vi "HitrapGUI.HTLE_TR5.vi"() -> ()   [LabVIEW 2014, in "HitrapGUI.lvlib"]
uses:
  HitrapGUI.lvlib
  CSlibraries/GUILib/GUILib.userEventsMainType.ctl
  CSlibraries-extern/DimLVEvent/DimIndicators/DimIndicators.anyType.ctl
  CSlibraries/GUILib/GUILib.simpleNumeric.ctl
  CSlibraries/GUILib/GUILib.basicNumeric.ctl
  CSlibraries-extern/DimLVEvent/DimIndicators/DimIndicators.numericType.ctl
  CSlibraries/UtilityLib/UtilityLib.valueStatus.ctl
  CS_Core/CSSystem/CoreDefs/CoreDefs.rawDataType.ctl
  CS_Core/CSSystem/CoreLib/CoreLib.double 2 byte array.vi
  CS_Core/CSSystem/CoreLib/CoreLib.int 2 byte array.vi
  CSlibraries/UtilityLib/UtilityLib.lvlib
  CS_Core/CSSystem/CSSystemLib/CSSystemLib.lvlib
  CSlibraries-extern/DimLVEvent/DimIndicators/DimIndicators.lvlib
  CS_Core/GUIs/GOGControllerGUI/GOGControllerGUI.lvlib
  CSlibraries/GUILib/GUILib.lvlib
  CS_Core/CSSystem/CoreLib/CoreLib.lvlib
  CSlibraries-extern/DimLVEvent/LVDimInterface/LVDimInterface.lvlib
panel:
  in  "MotorActivityLink-Act":T1
  in  "MotorLink-Act":T1
  in  "TR5DK1Link":T2
  in  "TR5DK2Link":T2
  in  "TR5DK1Ctl":T3 caption="TR5DK1" {"Progress Slide" scale=0.0..100.0; "Nom_Position" items=["Undefined", "Open", "Faraday Cup", "MCP"]}
  in  "TR5DK2Ctl":T3 caption="TR5DK2" {"Progress Slide" scale=0.0..100.0; "Nom_Position" items=["Undefined", "Open", "Faraday Cup", "MCP"]}
  in  "userEventsMain 2":T4
  in  "Next":bool
  in  "EnAn_TOF":bool=TRUE
  in  "EnAn_LEBT2":bool=TRUE
  in  "EnAn_LEBT1":bool=TRUE
  in  "EnAn_RFQ":bool=TRUE
  in  "EnAn_IH":bool=TRUE
  in  "EnAn_TOFCtl":T5 {"nom" step=1.0}
  in  "EnAn_LEBT2Ctl":T5 {"nom" step=1.0}
  in  "EnAn_LEBT1Ctl":T5 {"nom" step=1.0}
  in  "EnAn_RFQCtl":T5 {"nom" step=1.0}
  in  "EnAn_IHCtl":T5 {"nom" step=1.0}
  in  "TR3BB_2":bool=TRUE
  in  "TR3BB_1":bool=TRUE
  in  "TR3BB_2Ctl":T5 {"nom" step=1.0}
  in  "TR3BB_1Ctl":T5 {"nom" step=1.0}
  in  "TR5KY6Ctl":T5 {"nom" step=1.0}
  in  "TR5KX6Ctl":T5 {"nom" step=1.0}
  in  "TR5KY5Ctl":T5 {"nom" step=1.0}
  in  "TR5KX5Ctl":T5 {"nom" step=1.0}
  in  "TR5KY4Ctl":T5 {"nom" step=1.0}
  in  "TR5KX4Ctl":T5 {"nom" step=1.0}
  in  "TR5ME6Ctl":T5 {"nom" step=1.0}
  in  "TR5ME5Ctl":T5 {"nom" step=1.0}
  in  "TR5ME4Ctl":T5 {"nom" step=1.0}
  in  "TR5KY6":bool=TRUE
  in  "TR5KX6":bool=TRUE
  in  "TR5ME6":bool=TRUE
  in  "TR5ME5":bool=TRUE
  in  "TR5KY5":bool=TRUE
  in  "TR5KX5":bool=TRUE
  in  "TR5ME4":bool=TRUE
  in  "TR5KY4":bool=TRUE
  in  "TR5KX4":bool=TRUE
  in  "TR5ME3":bool=TRUE
  in  "TR5KY3":bool=TRUE
  in  "TR5KX3":bool=TRUE
  in  "TR5ME3Ctl":T5 {"nom" step=1.0}
  in  "TR5KY3Ctl":T5 {"nom" step=1.0}
  in  "TR5KX3Ctl":T5 {"nom" step=1.0}
  in  "TR5ME2Ctl":T5 {"nom" step=1.0}
  in  "TR5KY2Ctl":T5 {"nom" step=1.0}
  in  "TR5KX2Ctl":T5 {"nom" step=1.0}
  in  "TR5KY1Ctl":T5 {"nom" step=1.0}
  in  "TR5KX1Ctl":T5 {"nom" step=1.0}
  in  "TR5ME1Ctl":T5 {"nom" step=1.0}
  in  "TR5ME2":bool=TRUE
  in  "TR5KY2":bool=TRUE
  in  "TR5KX2":bool=TRUE
  in  "TR5KY1":bool=TRUE
  in  "TR5KX1":bool=TRUE
  in  "TR5ME1":bool=TRUE
  out "subSystem1State":string
  in  "subSystem1":bool
  out "subSystem1StateQuality":string
  in  "subControllersIgnoredDIM":T1
  in  "iniData":string
  in  "stop":bool
  in  "dummy":bool
  in  "parentSystem":bool
  in  "userEvent":refnum<user-event>
  # "TR5"
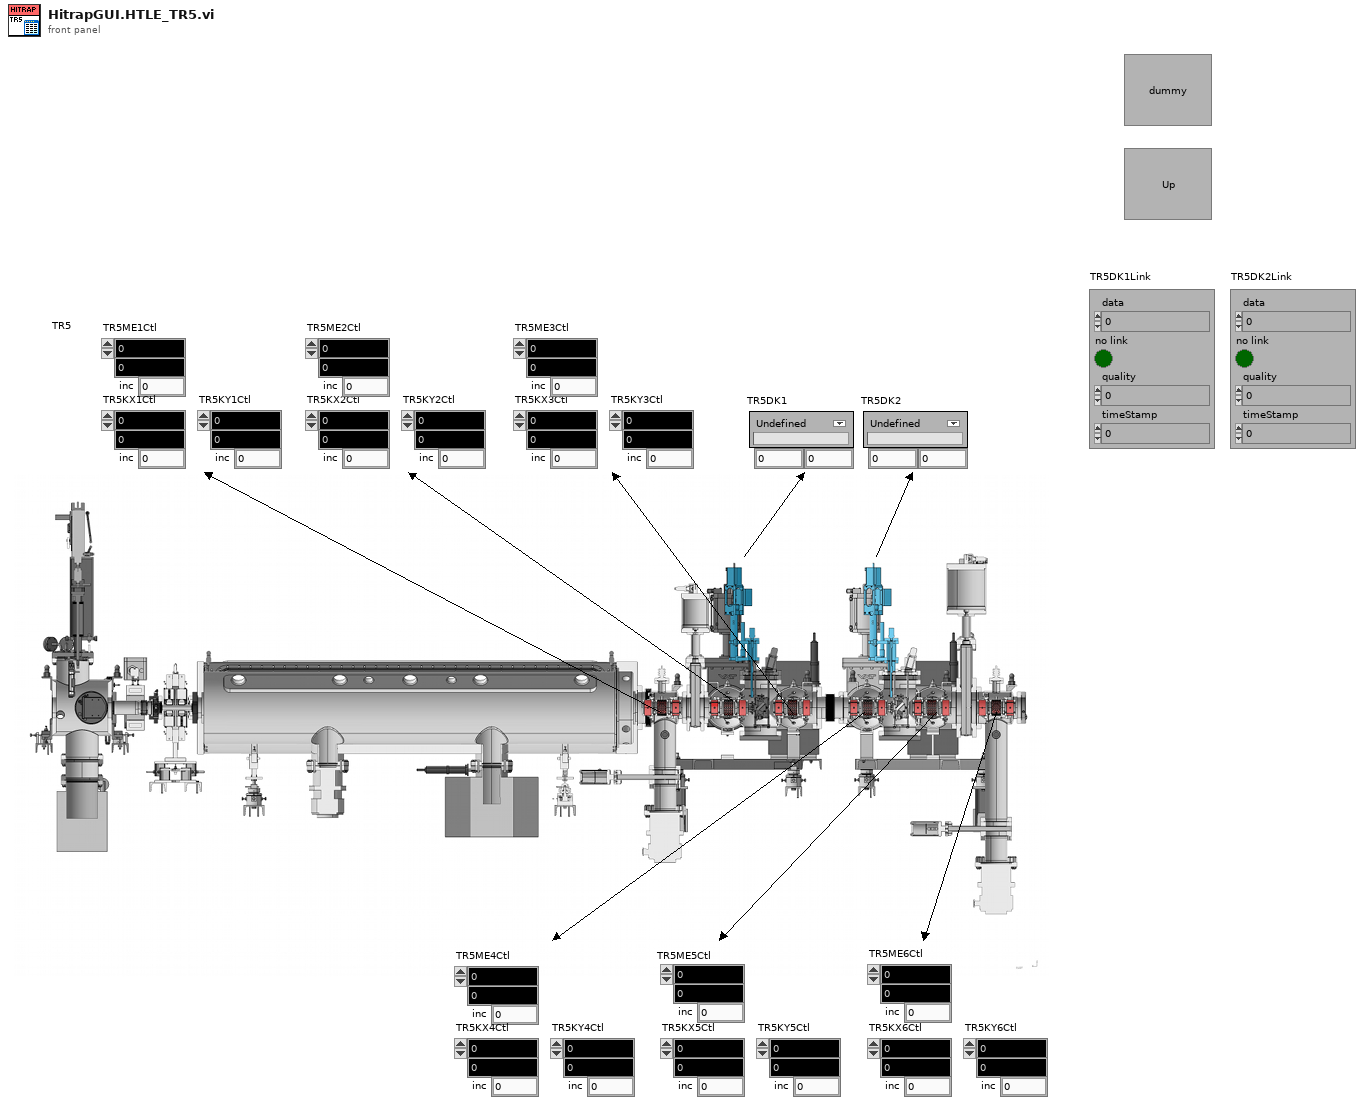
[diagram p1: front panel]
types:
  T1 = typedef "DimIndicators.lvlib/DimIndicators.anyType.ctl" = cluster{"data":string, "no link":bool, "quality":i32, "timeStamp":dbl}
  T2 = typedef "DimIndicators.lvlib/DimIndicators.numericType.ctl" = cluster{"data":dbl, "no link":bool, "quality":i32, "timeStamp":dbl}
  T3 = cluster{"Nom_Position":u8, "Progress Slide":u8, "TR6DK2Act":dbl, "TR6DK2Nom":dbl}
  T4 = typedef "GUILib.lvlib/GUILib.userEventsMainType.ctl" = cluster{"data":string, "dataType":i32}
  T5 = typedef "GUILib.lvlib/GUILib.simpleNumeric.ctl" = cluster{"nom":T6, "act":dbl, "inc":dbl}
  T6 = typedef "GUILib.lvlib/GUILib.basicNumeric.ctl" = dbl
  T7 = enum16{"Idle", "StartMotorActivity", "NewMotorDIM", "StopMotorActivity", "Stop"}
  T8 = typedef "UtilityLib.lvlib/UtilityLib.valueStatus.ctl" = enum16{"no info available", "stand by/off", "on", "warning", "alarm/malfunction", "not implemented", "user action required", "important information", "system default", "control default", "indicator default", "button default"}
  T9 = typedef "CoreDefs.rawDataType.ctl" = i8[]
  T10 = enum8{"Enabled", "Disabled", "Disabled and Grayed Out"}
  T11 = typedef "lveventtype.ctl" = enum32{"Null", "Timeout", "Annotation Menu Selection", "Annotation Menu Selection?", "App Instance Close", "App Instance Close?", "Autoscale Range Change", "Bookmark Info Change", "Cell Edit", "Cell Edit?", "Cursor Grab", "Cursor Grab?", "Cursor Menu Selection", "Cursor Menu Selection?", "Cursor Move", "Cursor Release", "Data Change", "Direction Change", "Display State Change", "Drag Ended", "Drag Enter", "Drag Leave", "Drag Over", "Drag Source Update", "Drag Starting", "Drag Starting?", "Drop", "Exec State Change", "Key Down", "Key Down?", "Key Repeat", "Key Repeat?", "Key Up", "Listbox Double Click", "Menu Activation?", "Menu Selection (App)", "Menu Selection? (App)", "Menu Selection (User)", "Mouse Down", "Mouse Down?", "Mouse Enter", "Mouse Leave", "Mouse Move", "Mouse Up", "Mouse Wheel", "NI Security User Change (App)", "Pane Size", "Panel Close", "Panel Close?", "Panel Resize", "Plot Attribute Change", "Scale Range Change", "Shortcut Menu Activation?", "Shortcut Menu Selection (App)", "Shortcut Menu Selection? (App)", "Shortcut Menu Selection (User)", "Tree Double Click", "Tree Drag", "Tree Drag?", "Tree Drop", "Tree Drop?", "Tree Item Close", "Tree Item Close?", "Tree Item Open", "Tree Item Open?", "User Event", "Value Change"}
  T12 = cluster{"TR5DK1Ctl":refnum<vi>, "byteArray out":T9}
  T13 = typedef "HitrapGUI.lvlib/HitrapGUI.i attribute.ctl" = cluster{"SVs":refnum<k21>[], "DSCIntProc":string, "MotorActivityID":i32}
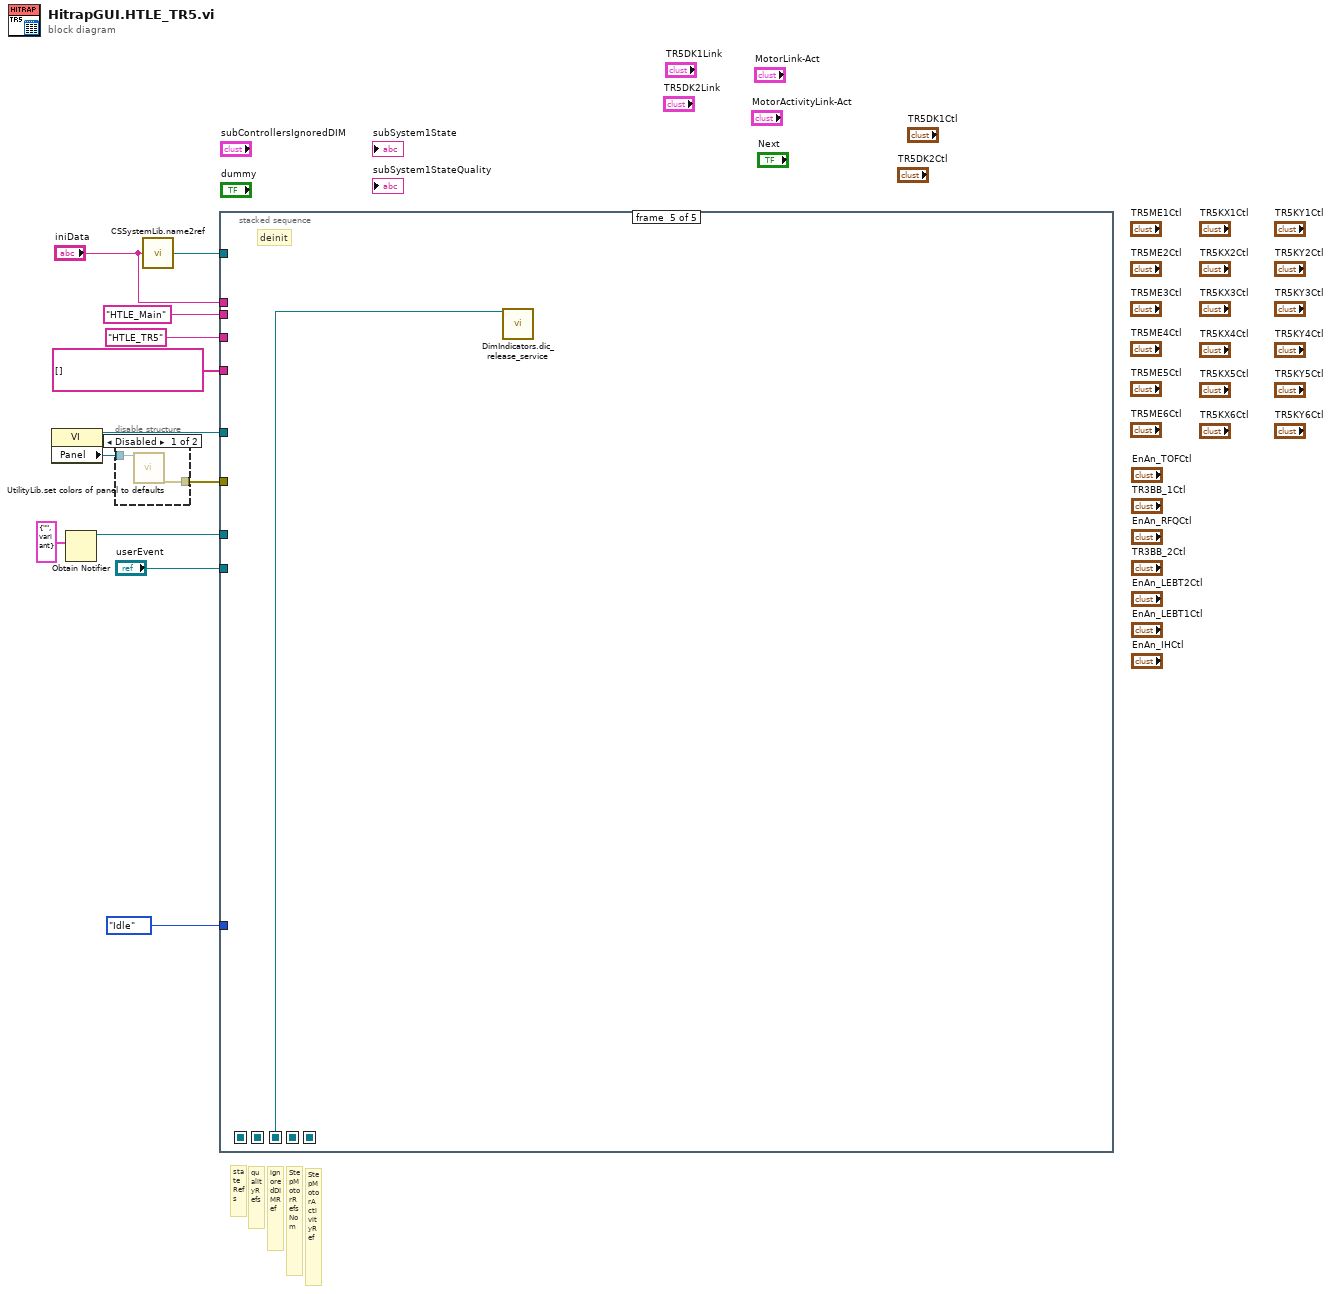
[diagram p0: block diagram]
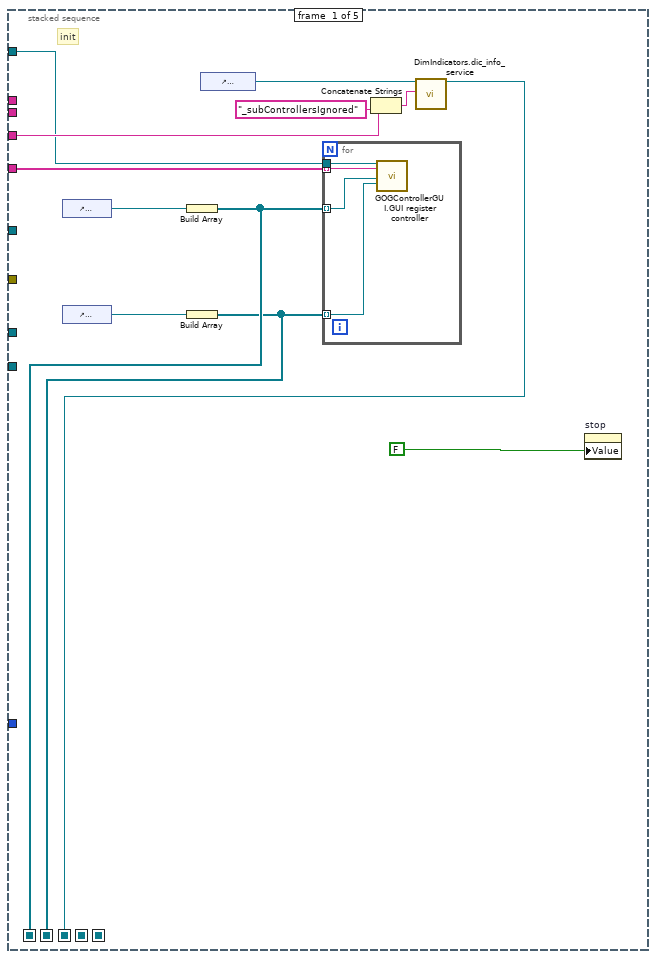
[diagram p3: hidden frame]
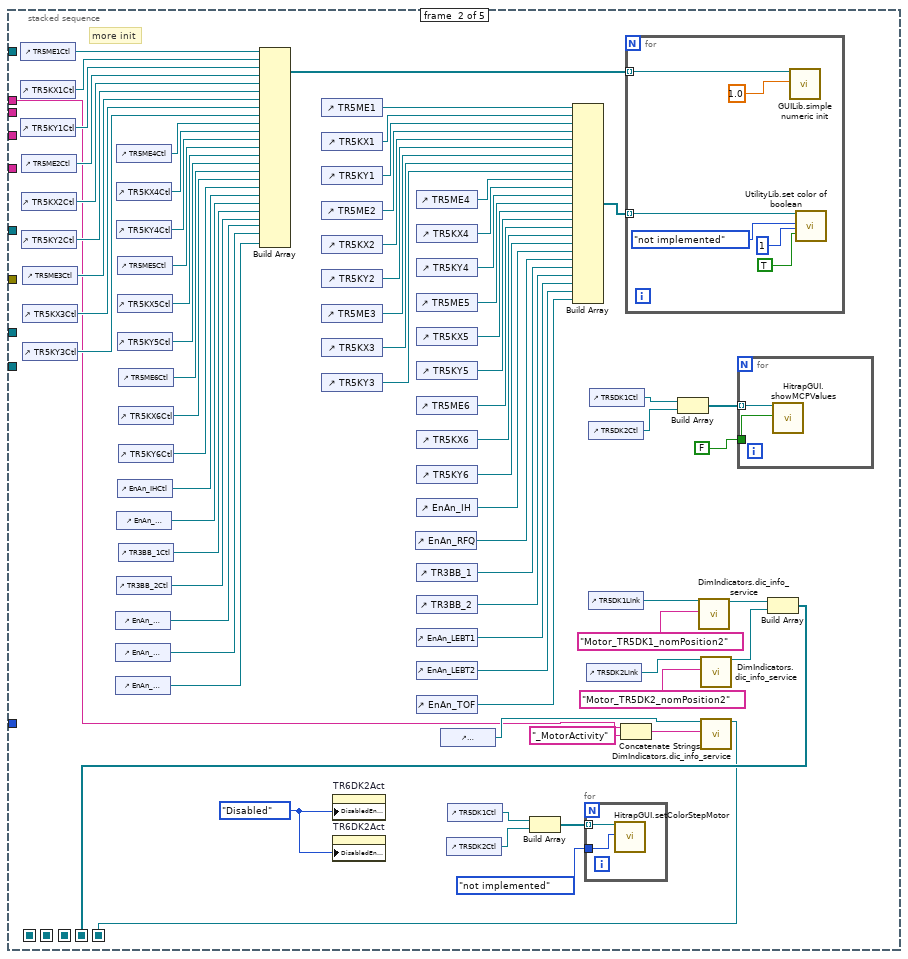
[diagram p4: hidden frame]
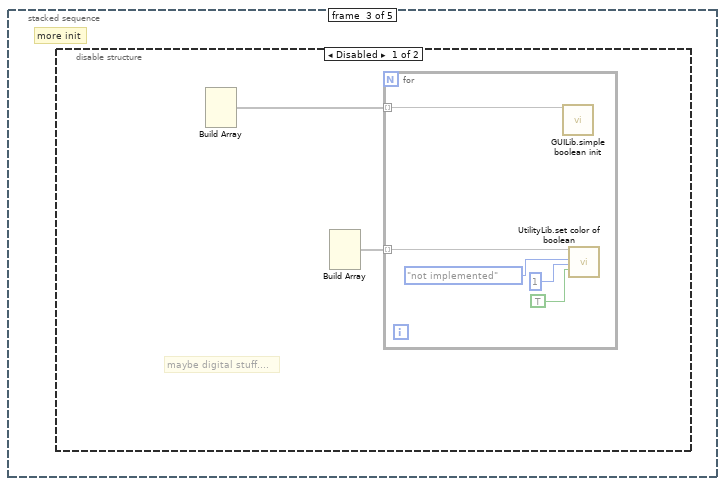
[diagram p5: hidden frame]
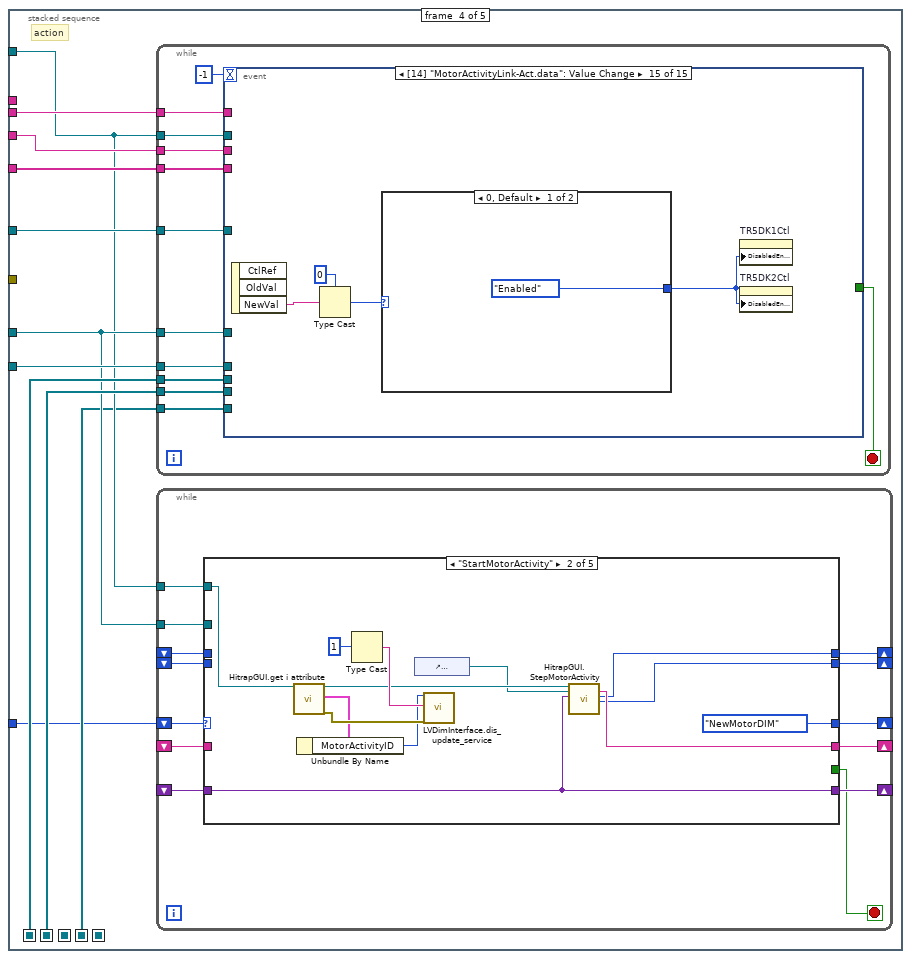
[diagram p7: hidden frame]
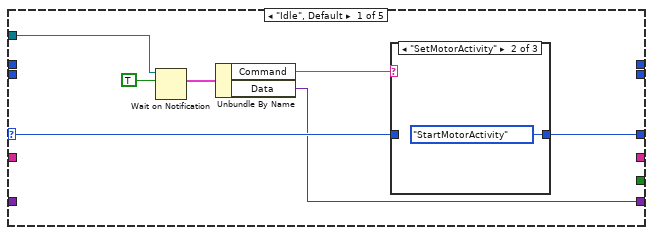
[diagram p8: hidden frame]
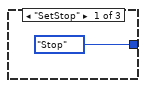
[diagram p9: hidden frame]
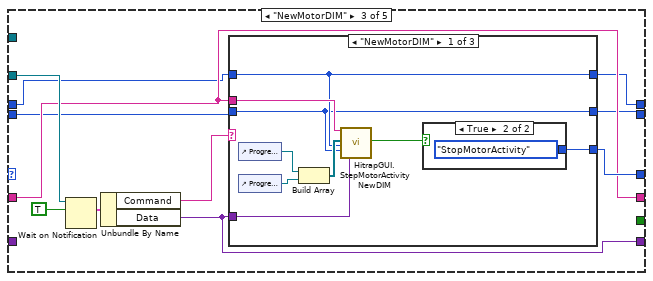
[diagram p11: hidden frame]
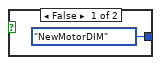
[diagram p12: hidden frame]
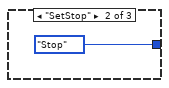
[diagram p13: hidden frame]
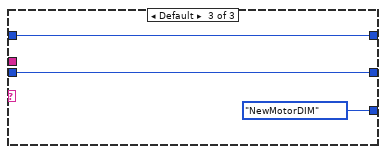
[diagram p14: hidden frame]
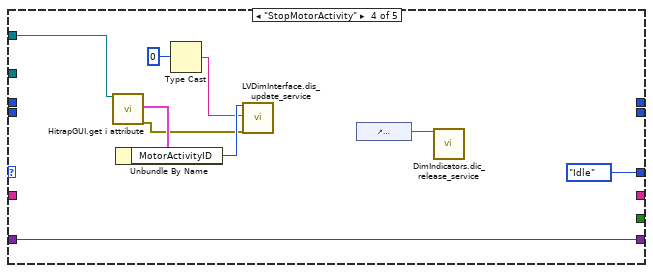
[diagram p15: hidden frame]
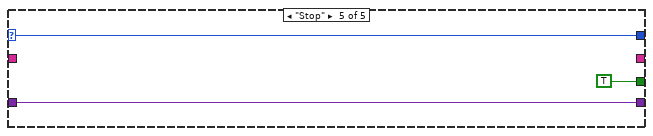
[diagram p16: hidden frame]
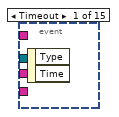
[diagram p17: hidden frame]
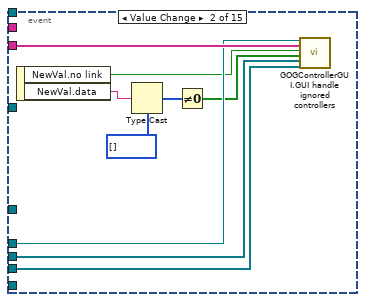
[diagram p18: hidden frame]
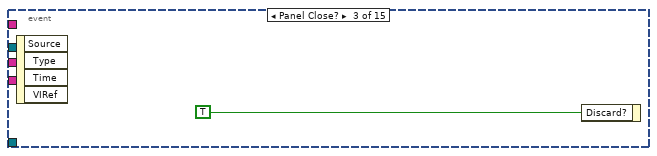
[diagram p19: hidden frame]
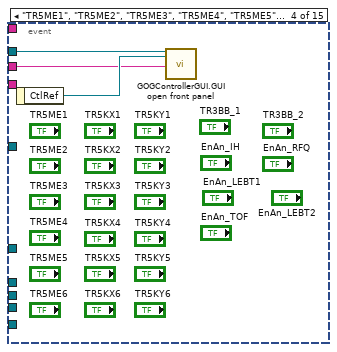
[diagram p20: hidden frame]
diagram:
  # "StepMotorActivityRef"
  # "StepMotorRefsNom"
  # "qualityRefs"
  # "ignoredDIMRef"
  # "stateRefs"
  n1 = property class="VI"() -> (reference out=w10:refnum<vi>, "Panel"=w11:refnum<vi>)  [unwired: 2 in, 1 out]
  n2 = Obtain Notifier(notification data type=cluster{"Command":string, "Data":variant} {"Command"="", "Data"=variant} ("EventData")) -> (notifier out=w2:refnum<notifier>)  [unwired: 3 in, 2 out]
  n3 = disable-structure shown="Disabled" {
    disable-tunnel: w11 -> [w14 _]
    disable-tunnel: [w13 _] -> w9
    frame Disabled {
      n4 = call "UtilityLib.set colors of panel to defaults.vi"("Front Panel"=w14) -> ("error out"=w13:errorcluster)  [unwired: 18 in]
    }
    frame Enabled {
    }
  }
  n5 = call "CSSystemLib.name2ref.vi"("name"="iniData") -> ("obj refnum"=w6:refnum<vi>)
  n6 = stacked-sequence {
    seq-local: [w16 _ _ _ _] -> [_ _ _ _ w346]
    seq-local: [w17 _ _ _ _] -> [_ _ _ w138 _]
    seq-local: [w15 _ _ _ _] -> [_ _ _ w137 _]
    seq-local: [_ w37 _ _ _] -> [_ _ _ w132 _]
    seq-local: [_ w36 _ _ _] -> [_ _ _ _ _]
    tunnel: "userEvent" -> [_ _ _ w141 _]
    tunnel: w10 -> [_ _ _ w140 _]
    tunnel: w9 -> [_ _ _ _ _]
    tunnel: "HTLE_TR5" -> [w22 _ _ w136 _]
    tunnel: string[] [] -> [w21 _ _ w139 _]
    tunnel: w6 -> [w20 _ _ w133 _]
    tunnel: "HTLE_Main" -> [_ _ _ w135 _]
    tunnel: "iniData" -> [_ w38 _ _ _]
    tunnel: w2 -> [_ _ _ w134 _]
    tunnel: T7."Idle" -> [_ _ _ w131 _]
    frame #0 {
      # "init"
      n7 = control-ref of="dummySubSystemState"() -> (w19:refnum<vi>)
      n8 = control-ref of="dummySubSystemStateQuality"() -> (w18:refnum<vi>)
      n9 = Build Array(w19) -> (w17:refnum<vi>[])
      n10 = Build Array(w18) -> (w15:refnum<vi>[])
      n11 = control-ref of="subControllersIgnoredDIM"() -> (w23:refnum<vi>)
      n12 = for {
        tunnel: w17 -> [w30] mode=indexing
        tunnel: w21 -> [w28] mode=indexing
        tunnel: w15 -> [w27] mode=indexing
        tunnel: w20 -> [w29]
        n13 = call "GOGControllerGUI.GUI register controller.vi"("i ref in"=w29, "controllerName"=w28, "subSystemState"=w30, "subSystemStateQuality"=w27) -> ()  [unwired: 14 in, 2 out]
      }
      n14 = Concatenate Strings(w22, "_subControllersIgnored" ("string")) -> (w25:string)
      n15 = call "DimIndicators.dic_info_service.vi"("controlRef"=w23, "serviceName"=w25) -> ("controlRef out"=w16:refnum<vi>)  [unwired: 16 in, 1 out]
      n16 = property on="stop" class="Bool (strict)"("Value"=FALSE ("stop")) -> ()  [unwired: 2 in, 2 out]
    }
    frame #1 {
      w31 = T10."Disabled" ("Disabled")
      # "more init"
      n17 = control-ref of="TR5ME1Ctl"() -> (w103:refnum<vi>)
      n18 = control-ref of="TR5KX1Ctl"() -> (w102:refnum<vi>)
      n19 = control-ref of="TR5KY1Ctl"() -> (w101:refnum<vi>)
      n20 = control-ref of="TR5ME2Ctl"() -> (w96:refnum<vi>)
      n21 = control-ref of="TR5KX2Ctl"() -> (w95:refnum<vi>)
      n22 = control-ref of="TR5KY2Ctl"() -> (w94:refnum<vi>)
      n23 = control-ref of="TR5ME3Ctl"() -> (w93:refnum<vi>)
      n24 = control-ref of="TR5KX3Ctl"() -> (w92:refnum<vi>)
      n25 = control-ref of="TR5KY3Ctl"() -> (w91:refnum<vi>)
      n26 = control-ref of="EnAn_LEBT1Ctl"() -> (w57:refnum<vi>)
      n27 = control-ref of="EnAn_LEBT2Ctl"() -> (w56:refnum<vi>)
      n28 = control-ref of="EnAn_TOFCtl"() -> (w55:refnum<vi>)
      n29 = control-ref of="TR5ME4Ctl"() -> (w90:refnum<vi>)
      n30 = control-ref of="TR5KX4Ctl"() -> (w89:refnum<vi>)
      n31 = control-ref of="TR5KY4Ctl"() -> (w88:refnum<vi>)
      n32 = control-ref of="EnAn_RFQCtl"() -> (w64:refnum<vi>)
      n33 = control-ref of="TR3BB_2Ctl"() -> (w60:refnum<vi>)
      n34 = control-ref of="TR5ME5Ctl"() -> (w87:refnum<vi>)
      n35 = control-ref of="TR5KX5Ctl"() -> (w86:refnum<vi>)
      n36 = control-ref of="TR5KY5Ctl"() -> (w85:refnum<vi>)
      n37 = control-ref of="EnAn_IHCtl"() -> (w65:refnum<vi>)
      n38 = control-ref of="TR5ME6Ctl"() -> (w84:refnum<vi>)
      n39 = control-ref of="TR5KX6Ctl"() -> (w83:refnum<vi>)
      n40 = control-ref of="TR5KY6Ctl"() -> (w82:refnum<vi>)
      n41 = control-ref of="TR3BB_1Ctl"() -> (w61:refnum<vi>)
      n42 = Build Array(w103, w102, w101, w96, w95, w94, w93, w92, w91, w90, w89, w88, w87, w86, w85, w84, w83, w82, w65, w64, w61, w60, w57, w56, w55) -> (w100:refnum<vi>[])
      n43 = control-ref of="TR5ME1"() -> (w99:refnum<vi>)
      n44 = control-ref of="TR5KX1"() -> (w98:refnum<vi>)
      n45 = control-ref of="TR5KY1"() -> (w81:refnum<vi>)
      n46 = control-ref of="TR5ME2"() -> (w80:refnum<vi>)
      n47 = control-ref of="TR5KX2"() -> (w79:refnum<vi>)
      n48 = control-ref of="TR5KY2"() -> (w78:refnum<vi>)
      n49 = control-ref of="TR5ME3"() -> (w77:refnum<vi>)
      n50 = control-ref of="TR5KX3"() -> (w76:refnum<vi>)
      n51 = control-ref of="TR5KY3"() -> (w75:refnum<vi>)
      n52 = property on="TR6DK2Act" class="DigNum (strict)"("DisabledEnum"=w31) -> ()  [unwired: 2 in, 2 out]
      n53 = property on="TR6DK2Act" class="DigNum (strict)"("DisabledEnum"=w31) -> ()  [unwired: 2 in, 2 out]
      n54 = control-ref of="EnAn_RFQ"() -> (w62:refnum<vi>)
      n55 = control-ref of="TR5ME4"() -> (w74:refnum<vi>)
      n56 = control-ref of="TR5KX4"() -> (w73:refnum<vi>)
      n57 = control-ref of="TR5KY4"() -> (w72:refnum<vi>)
      n58 = control-ref of="TR5ME5"() -> (w71:refnum<vi>)
      n59 = control-ref of="TR5KX5"() -> (w70:refnum<vi>)
      n60 = control-ref of="TR5KY5"() -> (w69:refnum<vi>)
      n61 = control-ref of="TR5ME6"() -> (w68:refnum<vi>)
      n62 = control-ref of="TR5KX6"() -> (w67:refnum<vi>)
      n63 = control-ref of="TR5KY6"() -> (w66:refnum<vi>)
      n64 = control-ref of="EnAn_IH"() -> (w63:refnum<vi>)
      n65 = control-ref of="TR3BB_1"() -> (w59:refnum<vi>)
      n66 = control-ref of="TR3BB_2"() -> (w58:refnum<vi>)
      n67 = control-ref of="EnAn_LEBT1"() -> (w54:refnum<vi>)
      n68 = control-ref of="EnAn_LEBT2"() -> (w53:refnum<vi>)
      n69 = control-ref of="EnAn_TOF"() -> (w52:refnum<vi>)
      n70 = control-ref of="MotorActivityLink-Act"() -> (w39:refnum<vi>)
      n71 = control-ref of="TR5DK2Ctl"() -> (w32:refnum<vi>)
      n72 = control-ref of="TR5DK1Ctl"() -> (w33:refnum<vi>)
      n73 = Build Array(w33, w32) -> (w34:refnum<vi>[])
      n74 = Build Array(w99, w98, w81, w80, w79, w78, w77, w76, w75, w74, w73, w72, w71, w70, w69, w68, w67, w66, w63, w62, w59, w58, w54, w53, w52) -> (w97:refnum<vi>[])
      n75 = for {
        tunnel: w34 -> [w105] mode=indexing
        tunnel: UtilityLib.valueStatus."not implemented" ("State") -> [w104]
        n76 = call "HitrapGUI.setColorStepMotor.vi"("Cluster Refnum"=w105, "State"=w104) -> ()  [unwired: 16 in, 2 out]
      }
      n77 = control-ref of="TR5DK2Link"() -> (w40:refnum<vi>)
      n78 = control-ref of="TR5DK2Ctl"() -> (w48:refnum<vi>)
      n79 = control-ref of="TR5DK1Link"() -> (w41:refnum<vi>)
      n80 = control-ref of="TR5DK1Ctl"() -> (w49:refnum<vi>)
      n81 = Concatenate Strings(w38, "_MotorActivity" ("string")) -> (w46:string)
      n82 = for {
        tunnel: w100 -> [w113] mode=indexing
        tunnel: w97 -> [w109] mode=indexing
        n83 = call "GUILib.simple numeric init.vi"("ctlRef"=w113, "increment"=1.0) -> ()  [unwired: 16 in, 2 out]
        n84 = call "UtilityLib.set color of boolean.vi"("button"=w109, "valueStatus"=UtilityLib.valueStatus."not implemented", "nOfPair (0)"=1, "setTRUEColor (FALSE)"=TRUE) -> ()  [unwired: 15 in, 1 out]
      }
      n85 = Build Array(w49, w48) -> (w50:refnum<vi>[])
      n86 = call "DimIndicators.dic_info_service.vi"("controlRef"=w41, "serviceName"="Motor_TR5DK1_nomPosition2") -> ("controlRef out"=w42:refnum<vi>)  [unwired: 16 in, 1 out]
      n87 = call "DimIndicators.dic_info_service.vi"("controlRef"=w40, "serviceName"="Motor_TR5DK2_nomPosition2") -> ("controlRef out"=w45:refnum<vi>)  [unwired: 16 in, 1 out]
      n88 = call "DimIndicators.dic_info_service.vi"("controlRef"=w39, "serviceName"=w46) -> ("controlRef out"=w36:refnum<vi>)  [unwired: 16 in, 1 out]
      n89 = for {
        tunnel: w50 -> [w107] mode=indexing
        tunnel: FALSE ("Visible") -> [w106]
        n90 = call "HitrapGUI.showMCPValues.vi"("Cluster Refnum"=w107, "show"=w106) -> ()  [unwired: 16 in, 2 out]
      }
      n91 = Build Array(w42, w45) -> (w37:refnum<vi>[])
    }
    frame #2 {
      # "more init"
      n92 = disable-structure shown="Disabled" {
        frame Disabled {
          # "maybe digital stuff...."
          n93 = Build Array() -> (w120:void[], w125:dbl, w124:dbl, w123:dbl, w122:dbl, w121:dbl)
          n94 = Build Array() -> (w114:void[], w119:dbl, w118:dbl, w117:dbl, w116:dbl, w115:dbl)
          n95 = for {
            tunnel: w120 -> [w130] mode=indexing
            tunnel: w114 -> [w126] mode=indexing
            n96 = call "GUILib.simple boolean init.vi"("ctlRef"=w130) -> ()  [unwired: 17 in, 2 out]
            n97 = call "UtilityLib.set color of boolean.vi"("button"=w126, "valueStatus"=UtilityLib.valueStatus."not implemented", "nOfPair (0)"=1, "setTRUEColor (FALSE)"=TRUE) -> ()  [unwired: 15 in, 1 out]
          }
        }
        frame Enabled {
        }
      }
    }
    frame #3 {
      # "action"
      n98 = while {
        tunnel: w141 -> [w227]
        tunnel: w140 -> [w225]
        tunnel: w139 -> [w223]
        tunnel: w138 -> [w222]
        tunnel: w137 -> [w221]
        tunnel: w133 -> [w220]
        tunnel: w136 -> [w219]
        tunnel: w135 -> [w218]
        tunnel: w134 -> [w217]
        tunnel: w132 -> [w216]
        stop <- w224 stop-if-true
        n99 = event shown="[14] \"MotorActivityLink-Act.data\": Value Change" {
          selector: _ -> [_ _ _ _ _ _ _ _ _ _ _ _ _ _ _]
          dyn-events: _ -> [_ _ _ _ _ _ _ _ _ _ _ _ _ _ _]
          timeout: -1 -> [_ _ _ _ _ _ _ _ _ _ _ _ _ _ _]
          tunnel: w227 -> [_ w232 _ _ w241 w252 _ w261 w265 _ _ _ _ _ _]
          tunnel: w225 -> [_ _ _ _ _ _ _ _ _ _ _ _ _ _ _]
          tunnel: [_ _ _ _ _ _ _ _ _ "stop" _ _ _ _ _] -> w224
          tunnel: w223 -> [_ w233 _ _ _ w248 _ _ _ _ _ _ _ _ _]
          tunnel: w222 -> [_ w229 _ _ _ _ _ _ _ _ _ _ _ _ _]
          tunnel: w221 -> [_ w228 _ _ _ _ _ _ _ _ _ _ _ _ _]
          tunnel: w220 -> [_ _ _ w240 _ _ _ _ w269 _ _ _ _ _ _]
          tunnel: w219 -> [_ _ _ w238 _ _ _ w259 w263 _ _ _ _ _ _]
          tunnel: w218 -> [_ _ _ _ _ w247 _ _ _ _ _ _ _ _ _]
          tunnel: w217 -> [_ _ _ _ _ _ _ _ _ w270 _ _ w312 w332 _]
          tunnel: w216 -> [_ _ _ _ _ _ _ _ _ _ w277 _ _ _ _]
          event Timeout {
            n100 = event-data() -> ()  [unwired: 1 in, 2 out]
          }
          event Value Change {
            n101 = event-data() -> ("NewVal.no link"=w231:bool, "NewVal.data"=w234:string)  [unwired: 1 in]
            n102 = Type Cast(type=T9 [] ("Array"), x=w234) -> (*(type *) &x=w236:T9)
            n103 = Not Equal To 0?(x=w236) -> (x != 0?=w230:bool[])
            n104 = call "GOGControllerGUI.GUI handle ignored controllers.vi"("userEvent"=w232, "controllerNames"=w233, "NOLINK"=w231, "controllersIgnored"=w230, "stateRefs"=w229, "qualityRefs"=w228) -> ()  [unwired: 14 in]
          }
          event Panel Close? {
            n105 = event-data() -> ()  [unwired: 1 in, 4 out]
            n106 = event-data("Discard?"=TRUE) -> ()  [unwired: 1 in, 1 out]
          }
          event "TR5ME1", "TR5ME2", "TR5ME3", "TR5ME4", "TR5ME5", "TR5ME6", "TR5KX1", "TR5KX2", "TR5KX3", "TR5KX4", "TR5KX5", "TR5KX6", "TR5KY1", "TR5KY2", "TR5KY3", "TR5KY4", "TR5KY5", "TR5KY6", "EnAn_IH", "EnAn_RFQ", "TR3BB_1", "TR3BB_2", "EnAn_LEBT1", "EnAn_LEBT2", "EnAn_TOF": Value Change {
            n107 = event-data() -> ("CtlRef"=w239:refnum<vi>)  [unwired: 1 in]
            n108 = call "GOGControllerGUI.GUI open front panel.vi"("i ref in"=w240, "elementRef"=w239, "controller"=w238) -> ()  [unwired: 15 in, 2 out]
          }
          event "Next": Value Change {
            n109 = event-data() -> ()  [unwired: 1 in, 3 out]
            n110 = Bundle By Name(cluster="userEventsMain 2", "data"="HTLE_TR6BT1", "dataType"=0) -> (w245:T4)
            n111 = Generate User Event(user event=w241, event data cluster=w245) -> ()  [unwired: 2 in, 2 out]
          }
          event "subSystem1", "parentSystem": Value Change {
            n112 = event-data() -> ("CtlRef"=w250:refnum<vi>)  [unwired: 1 in]
            n113 = control-ref of="parentSystem"() -> (w249:refnum<vi>)
            n114 = control-ref of="subSystem1"() -> (w253:refnum<vi>)
            n115 = Build Array (concatenate)(w247, w248) -> (w246:string[])
            n116 = Build Array(w249, w253) -> (w251:refnum<vi>[])
            n117 = call "GOGControllerGUI.GUI set selected subcontroller.vi"("userEvent"=w252, "controllerNames"=w246, "controllerRefs"=w251, "controllerRef"=w250) -> ()  [unwired: 16 in]
          }
          event Value Change {
            n118 = event-data() -> ("CtlRef"=w255:refnum<vi>, "NewVal"=w254:dbl)  [unwired: 1 in]
            n119 = call "GUILib.simple numeric change increment.vi"("ctlRef"=w255, "increment"=w254) -> ()  [unwired: 16 in, 2 out]
          }
          event Mouse Enter; Mouse Leave {
            n120 = event-data() -> ("CtlRef"=w258:refnum<vi>, "Type"=w257:T11)  [unwired: 1 in]
            n121 = case shown="\"Mouse Enter\"" w257 {
              tunnel: [TRUE _] -> w256
              frame "Mouse Enter" {
              }
              frame Default {
              }
            }
            n122 = call "GUILib.simple numeric show increment.vi"("ctlRef"=w258, "show"=w256) -> ("error out"=w260:errorcluster)  [unwired: 16 in, 1 out]
            n123 = call "GOGControllerGUI.GUI set error.vi"("userEvent"=w261, "controller"=w259, "GUIError"=w260) -> ()  [unwired: 16 in, 1 out]
          }
          event Value Change {
            n124 = event-data() -> ("CtlRef"=w268:refnum<vi>, "NewVal"=w267:T6)  [unwired: 1 in]
            n125 = call-poly "CoreLib.data 2 byte array.vi"("f64"=w267) -> ("byteArray out"=w266:T9)  [unwired: 18 in]
            n126 = call "GOGControllerGUI.GUI set nominal value.vi"("i ref in"=w269, "nominalRef"=w268, "nominalData"=w266, "controller"=w263) -> ("error out"=w264:errorcluster)  [unwired: 14 in, 1 out]
            n127 = call "GOGControllerGUI.GUI set error.vi"("userEvent"=w265, "controller"=w263, "GUIError"=w264) -> ()  [unwired: 16 in, 1 out]
          }
          event "stop": Value Change {
            n128 = event-data() -> ()  [unwired: 1 in, 6 out]
            n129 = Bundle("SetStop", "Data"=variant) -> (w273:cluster{string, "Data":variant})  [unwired: 1 in]
            n130 = Send Notification(notification=w273, notifier=w270) -> ()  [unwired: 1 in, 2 out]
          }
          event Value Change {
            n131 = event-data() -> ("CtlRef"=w276:refnum<vi>, "NewVal.data"=w278:dbl, "NewVal.no link"=w275:bool)  [unwired: 1 in]
            n132 = case shown="-2" w278 {
              tunnel: [w306 -1.0] -> w280
              tunnel: w278 -> [w306 _]
              frame 0, Default {
              }
              frame -2 {
              }
            }
            n133 = Increment(x=w280) -> (x+1=w281:dbl)
            n134 = To Unsigned Byte Integer(number=w281) -> (unsigned 8bit integer=w279:u8)
            n135 = for {
              tunnel: w275 -> [w288]
              tunnel: w276 -> [w284]
              tunnel: w279 -> [w287]
              tunnel: w277 -> [w286] mode=indexing
              i -> [w289]
              w282 = 0
              n136 = Type Cast(type=w282, x=w286) -> (*(type *) &x=w285:i32)
              n137 = Type Cast(type=w282, x=w284) -> (*(type *) &x=w283:i32)
              n138 = Equal?(x=w283, y=w285) -> (x = y?=w290:bool)
              n139 = case shown="True" w290 {
                tunnel: w289 -> [_ w296]
                tunnel: w288 -> [_ w295]
                tunnel: w287 -> [_ w294]
                frame False {
                }
                frame True {
                  n140 = case shown="0" w296 {
                    tunnel: w294 -> [_ w303 w304]
                    tunnel: [_ w302 w305] -> w293
                    frame Default {
                    }
                    frame 0 {
                      n141 = property on="Nom_Position" class="Ring (strict)"("Value"=w303) -> ()  [unwired: 2 in, 2 out]
                      n142 = control-ref of="TR5DK1Ctl"() -> (w302:refnum<vi>)
                    }
                    frame 1 {
                      n143 = property on="Nom_Position" class="Ring (strict)"("Value"=w304) -> ()  [unwired: 2 in, 2 out]
                      n144 = control-ref of="TR5DK2Ctl"() -> (w305:refnum<vi>)
                    }
                  }
                  n145 = case shown="False" w295 {
                    tunnel: [w298 UtilityLib.valueStatus."not implemented" ("State")] -> w292
                    tunnel: TRUE -> [w297 _]
                    frame False {
                      n146 = case shown="False" w297 {
                        tunnel: [UtilityLib.valueStatus."warning" ("State") UtilityLib.valueStatus."on" ("State")] -> w298
                        frame False {
                        }
                        frame True {
                        }
                      }
                    }
                    frame True {
                    }
                  }
                  n147 = call "HitrapGUI.setColorStepMotor.vi"("Cluster Refnum"=w293, "State"=w292) -> ()  [unwired: 16 in, 2 out]
                }
              }
            }
          }
          event "TR5DK2Ctl", "TR5DK1Ctl": Mouse Enter; "TR5DK2Ctl", "TR5DK1Ctl": Mouse Leave {
            n148 = event-data() -> ("CtlRef"=w309:refnum<vi>, "Type"=w308:T11)  [unwired: 1 in]
            n149 = case shown="\"Mouse Enter\"" w308 {
              tunnel: [TRUE _] -> w310
              frame "Mouse Enter" {
              }
              frame Default {
              }
            }
            n150 = call "HitrapGUI.showMCPValues.vi"("Cluster Refnum"=w309, "show"=w310) -> ()  [unwired: 16 in, 2 out]
          }
          event "TR5DK1Ctl.Nom_Position", "TR5DK2Ctl.Nom_Position": Value Change {
            n151 = event-data() -> ("CtlRef"=w315:refnum<vi>, "NewVal"=w314:u8)  [unwired: 1 in, 1 out]
            n152 = Greater Than 0?(x=w314) -> (x > 0?=w313:bool)
            n153 = case shown="True" w313 {
              tunnel: w315 -> [_ w328]
              tunnel: w314 -> [_ w329]
              tunnel: w312 -> [_ w327]
              frame False {
              }
              frame True {
                n154 = Decrement(x=w329) -> (x-1=w320:u8)
                n155 = property class="Ring (strict)"(reference=w328) -> ("Owner"=w318:refnum<vi>)  [unwired: 1 in, 2 out]
                n156 = call-poly "CoreLib.data 2 byte array.vi"("i32"=0) -> ("byteArray out"=w322:T9)  [unwired: 18 in]
                n157 = call-poly "CoreLib.data 2 byte array.vi"("byteArray"=w322, "i32"=w320) -> ("byteArray out"=w319:T9)  [unwired: 17 in]
                n158 = control-ref of="TR5DK1Ctl"() -> (w316:refnum<vi>)
                n159 = To More Specific Class(target class=w316, reference=w318) -> (specific class reference=w317:refnum<vi>)  [unwired: 1 in, 1 out]
                n160 = Bundle("TR5DK1Ctl"=w317, "byteArray out"=w319) -> (w323:T12)  [unwired: 1 in]
                n161 = To Variant(anything=w323) -> (Variant=w324:variant)
                n162 = Bundle("SetMotorActivity", "Variant"=w324) -> (w326:cluster{string, "Variant":variant})  [unwired: 1 in]
                n163 = Send Notification(notification=w326, notifier=w327) -> ()  [unwired: 1 in, 2 out]
              }
            }
          }
          event Value Change {
            w338 = 0.0
            n164 = event-data() -> ("OldVal"=w330:string, "NewVal"=w331:string)  [unwired: 1 in, 1 out]
            n165 = Type Cast(type=w338, x=w331) -> (*(type *) &x=w339:dbl)
            n166 = Type Cast(type=w338, x=w330) -> (*(type *) &x=w337:dbl)
            n167 = Bundle(w337, w339) -> (w336:cluster{dbl, dbl})  [unwired: 1 in]
            n168 = To Variant(anything=w336) -> (Variant=w335:variant)
            n169 = Bundle("NewMotorDIM", "Variant"=w335) -> (w333:cluster{string, "Variant":variant})  [unwired: 1 in]
            n170 = Send Notification(notification=w333, notifier=w332) -> ()  [unwired: 1 in, 2 out]
          }
          event Value Change {
            n171 = event-data() -> ("NewVal"=w341:string)  [unwired: 1 in, 2 out]
            n172 = Type Cast(type=i16 0 ("x"), x=w341) -> (*(type *) &x=w342:i16)
            n173 = case shown="0, Default" w342 {
              tunnel: [T10."Enabled" ("Disabled") T10."Disabled and Grayed Out" ("Disabled")] -> w340
              frame 0, Default {
              }
              frame 1 {
              }
            }
            n174 = property on="TR5DK1Ctl" class="Clust (strict)"("DisabledEnum"=w340) -> ()  [unwired: 2 in, 2 out]
            n175 = property on="TR5DK2Ctl" class="Clust (strict)"("DisabledEnum"=w340) -> ()  [unwired: 2 in, 2 out]
          }
        }
      }
      n176 = while {
        tunnel: w134 -> [w151]
        tunnel: w133 -> [w152]
        shift-right: [w153] -> _
        shift-left: w131 -> [w154]
        shift-right: [w150] -> _
        shift-left: _ -> [w147]
        shift-right: [w149] -> _
        shift-left: _ -> [w148]
        shift-right: [w146] -> _
        shift-left: _ -> [w145]
        shift-right: [w143] -> _
        shift-left: _ -> [w142]
        stop <- w144 stop-if-true
        n177 = case shown="\"StartMotorActivity\"" w154 {
          selector: w154 -> [w158 _ _ _ w215]
          tunnel: w151 -> [w155 _ w185 _ _]
          tunnel: [w157 T7."NewMotorDIM" w184 T7."Idle" w215] -> w153
          tunnel: [w156 w170 w183 w205 w214] -> w146
          tunnel: w152 -> [_ w171 _ w206 _]
          tunnel: w145 -> [_ w170 _ w205 w214]
          tunnel: [_ w168 w182 _ _] -> w143
          tunnel: [_ w167 w179 _ _] -> w150
          tunnel: [_ w166 w178 _ _] -> w149
          tunnel: [_ _ _ _ TRUE] -> w144
          tunnel: w147 -> [_ _ w181 _ _]
          tunnel: w148 -> [_ _ w180 _ _]
          tunnel: w142 -> [_ _ w182 _ _]
          frame "Idle", Default {
            n178 = Wait on Notification(notifier=w155, ignore previous (F)=TRUE) -> (notification=w161:cluster{"Command":string, "Data":variant})  [unwired: 2 in, 3 out]
            n179 = Unbundle By Name(w161) -> ("Command"=w160:string, "Data"=w156:variant)
            n180 = case shown="\"SetMotorActivity\"" w160 {
              tunnel: w158 -> [_ _ w164]
              tunnel: [T7."Stop" T7."StartMotorActivity" w164] -> w157
              frame "SetStop" {
              }
              frame "SetMotorActivity" {
              }
              frame "Idle", Default {
              }
            }
          }
          frame "StartMotorActivity" {
            n181 = call "HitrapGUI.get i attribute.vi"("i ref in"=w171) -> ("i ref out"=w172:refnum<vi>, "i attribute"=w173:T13, "error out"=w175:errorcluster)  [unwired: 16 in]
            n182 = Unbundle By Name(w173) -> ("MotorActivityID"=w174:i32)
            n183 = Type Cast(x=i16 1) -> (*(type *) &x=w177:string)  [unwired: 1 in]
            n184 = control-ref of="MotorLink-Act"() -> (w165:refnum<vi>)
            n185 = call "LVDimInterface.dis_update_service.vi"("my_serviceID"=w174, "data"=w177, "error in (no error)"=w175) -> ()  [unwired: 14 in, 3 out]
            n186 = call "HitrapGUI.StepMotorActivity.vi"("i ref in"=w172, "DIMPositioncontrolRef"=w165, "Data"=w170) -> ("MotorName"=w168:string, "StartPosition"=w167:i32, "StopPosition"=w166:i32)  [unwired: 12 in, 2 out]
          }
          frame "NewMotorDIM" {
            n187 = Wait on Notification(notifier=w185, ignore previous (F)=TRUE) -> (notification=w187:cluster{"Command":string, "Data":variant})  [unwired: 2 in, 3 out]
            n188 = Unbundle By Name(w187) -> ("Command"=w188:string, "Data"=w183:variant)
            n189 = case shown="\"NewMotorDIM\"" w188 {
              tunnel: [w197 T7."Stop" T7."NewMotorDIM"] -> w184
              tunnel: w181 -> [w192 _ w202]
              tunnel: w180 -> [w191 _ w201]
              tunnel: w183 -> [w194 _ _]
              tunnel: w182 -> [w193 _ _]
              tunnel: [w192 _ w202] -> w179
              tunnel: [w191 _ w201] -> w178
              frame "NewMotorDIM" {
                n190 = control-ref of="Progress Slide"() -> (w189:refnum<vi>)
                n191 = control-ref of="Progress Slide"() -> (w190:refnum<vi>)
                n192 = Build Array(w189, w190) -> (w195:refnum<vi>[])
                n193 = call "HitrapGUI.StepMotorActivityNewDIM.vi"("MotorName"=w193, "Progress Slide Array"=w195, "StartPosition"=w192, "StopPosition"=w191, "Data"=w194) -> ("Finished?"=w196:bool)  [unwired: 12 in, 2 out]
                n194 = case shown="True" w196 {
                  tunnel: [T7."NewMotorDIM" T7."StopMotorActivity"] -> w197
                  frame False {
                  }
                  frame True {
                  }
                }
              }
              frame "SetStop" {
              }
              frame Default {
              }
            }
          }
          frame "StopMotorActivity" {
            n195 = call "HitrapGUI.get i attribute.vi"("i ref in"=w206) -> ("i attribute"=w211:T13, "error out"=w209:errorcluster)  [unwired: 16 in, 1 out]
            n196 = Unbundle By Name(w211) -> ("MotorActivityID"=w210:i32)
            n197 = Type Cast(x=i16 0) -> (*(type *) &x=w207:string)  [unwired: 1 in]
            n198 = call "LVDimInterface.dis_update_service.vi"("my_serviceID"=w210, "data"=w207, "error in (no error)"=w209) -> ()  [unwired: 14 in, 3 out]
            n199 = control-ref of="MotorLink-Act"() -> (w204:refnum<vi>)
            n200 = call "DimIndicators.dic_release_service.vi"("controlRef"=w204) -> ()  [unwired: 18 in, 1 out]
          }
          frame "Stop" {
          }
        }
      }
    }
    frame #4 {
      # "deinit"
      n201 = call "DimIndicators.dic_release_service.vi"("controlRef"=w346) -> ()  [unwired: 18 in, 1 out]
    }
  }
